vi "Prepare server URL (Optional).vi"(1 "server url in":string) -> (0 "server url out":string)   [LabVIEW 2020]
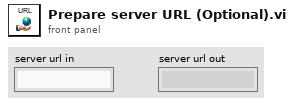
[diagram p1: front panel]
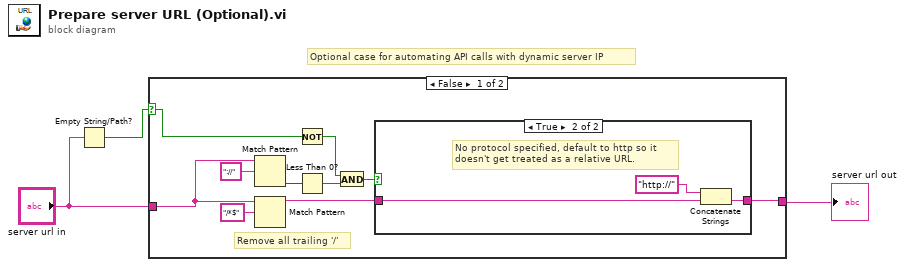
[diagram p0: block diagram]
diagram:
  # "Optional case for automating API calls with dynamic server IP"
  n1 = Empty String/Path?(string/path="server url in") -> (empty?=w3:bool)
  n2 = case shown="False" w3 {
    selector: w3 -> [w4 _]
    tunnel: [w8 w18] -> w1
    tunnel: "server url in" -> [w5 w18]
    frame False {
      # "Remove all trailing '/'"
      n3 = Match Pattern(string=w5, regular expression="://") -> (offset past match=w12:i32)  [unwired: 1 in, 3 out]
      n4 = Match Pattern(string=w5, regular expression="/*$") -> (before substring=w7:string)  [unwired: 1 in, 3 out]
      n5 = Not(x=w4) -> (.not. x?=w10:bool)
      n6 = Less Than 0?(x=w12) -> (x < 0?=w11:bool)
      n7 = And(x=w10, y=w11) -> (x .and. y?=w9:bool)
      n8 = case shown="True" w9 {
        tunnel: w7 -> [w14 w16]
        tunnel: [w14 w15] -> w8
        frame False {
          # "Protocol specified or using empty string to represent host server."
        }
        frame True {
          # "No protocol specified, default to http so it doesn't get treated as a relative URL."
          n9 = Concatenate Strings("http://" ("string"), w16) -> (w15:string)
        }
      }
    }
    frame True {
    }
  }
  "server url out" <- w1
